vi "Write Initialized.vi"(10 "Initialized (True)":bool=TRUE, 11 "Interlock in":refnum<class "Interlock.lvclass">) -> (3 "Interlock out":refnum<class "Interlock.lvclass">)   [LabVIEW 2015, in "Interlocks.lvlib" / "Interlock.lvclass"]
uses:
  Interlock.lvclass
  Interlock.lvclass/Interlock.ctl
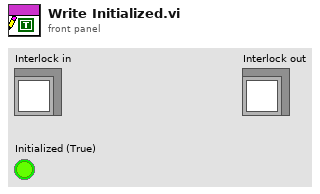
[diagram p1: front panel]
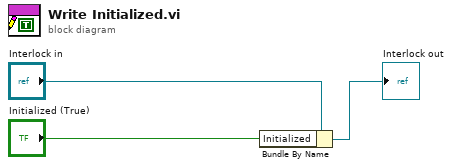
[diagram p0: block diagram]
diagram:
  n1 = Bundle By Name(cluster="Interlock in", "Initialized"="Initialized (True)") -> (→"Interlock out":refnum<class "Interlock.lvclass">)
